vi "getSeverNotifier.vi"(8 "error in (no error)":errorcluster, 10 "notifier timeout":i32, 11 "TcpServerCmd in":refnum<class "TcpServerCmd.lvclass">) -> (0 "error out":errorcluster, 1 "timeout?":bool, 2 "connStatusCluster":T1, 3 "TcpServerCmd out":refnum<class "TcpServerCmd.lvclass">)   [LabVIEW 2018, in "TcpServerCmd.lvclass"]
doc: "Get the notifier from TcpServerCmd.tcpServerStateMachine.vi. The notifier will inform the user if the command server disconnects or reconnects to the client. This vi is needed to avoid to expose the TcpServerBase.getServerNotifier.vi to the user."
uses:
  TcpServerCmd.lvclass
  home/pcortes/github/ts_labview_tcp_json/src/TcpServerBase/TcpServerBase.lvclass
  TcpServerBase/TcpServerBase.lvclass
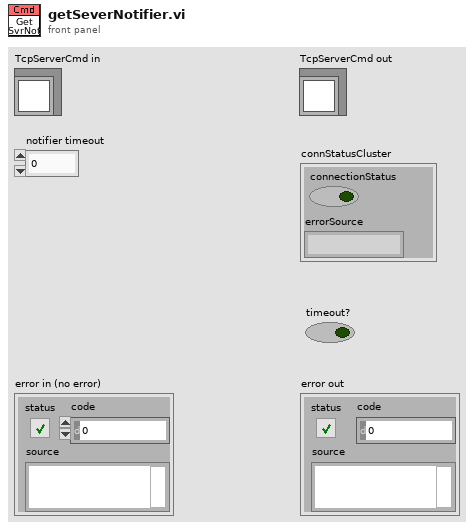
[diagram p1: front panel]
types:
  T1 = cluster{"connectionStatus":bool, "errorSource":string}
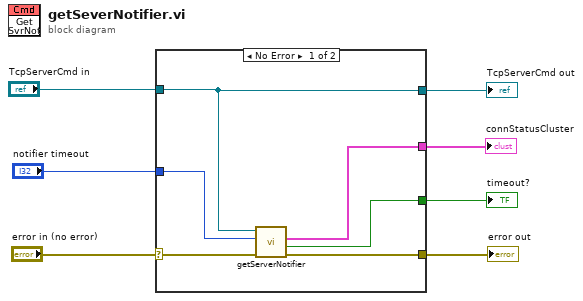
[diagram p0: block diagram]
diagram:
  n1 = case shown="No Error" "error in (no error)" {
    selector: "error in (no error)" -> [w13 w15]
    tunnel: "notifier timeout" -> [w12 _]
    tunnel: "TcpServerCmd in" -> [w8 w14]
    tunnel: [w9 w15] -> w4
    tunnel: [w11 _] -> w3
    tunnel: [w10 _] -> w2
    tunnel: [w8 w14] -> w1
    frame No Error {
      n2 = call "getServerNotifier.vi"("error in (no error)"=w13, "notifier timeout"=w12, "TcpServerBase in"=w8) -> ("error out"=w9:errorcluster, "timeout?"=w10:bool, "connStatusCluster"=w11:T1)  [unwired: 5 in, 1 out]
    }
    frame Error {
    }
  }
  "error out" <- w4
  "connStatusCluster" <- w3
  "timeout?" <- w2
  "TcpServerCmd out" <- w1
